vi "Init Dashboard Panel.vi"(8 "error in (no error)":errorcluster, 11 "SB App in":refnum<class "SB App.lvclass">) -> (0 "error out":errorcluster, 3 "SB App out":refnum<class "SB App.lvclass">)   [LabVIEW 2020, in "SB App.lvlib" / "SB App.lvclass"]
uses:
  SB App.lvclass
  Dashboard Panel/Dashboard Panel.lvclass
  C:/Program Files (x86)/National Instruments/LabVIEW 2020/vi.lib/IlluminatedG/IG OOPanel/OOPanel/Panel/Panel.lvclass
  SB App.lvclass/SB App.ctl
  <vilib>/IlluminatedG/IG OOPanel/OOPanel/Manager/Manager.lvclass
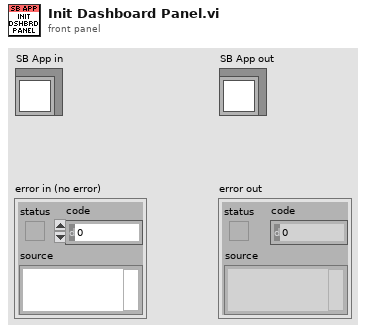
[diagram p1: front panel]
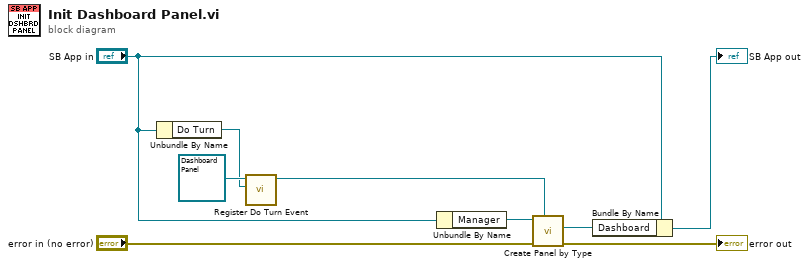
[diagram p0: block diagram]
diagram:
  n1 = Unbundle By Name("SB App in") -> ("Do Turn"=w5:refnum<user-event>)
  n2 = call "Register Do Turn Event.vi"("Do Turn"=w5, "Dashboard Panel in"=refnum<class "Dashboard Panel.lvclass"> refnum ("SB App.lvlib:Dashboard Panel.lvclass")) -> ("Dashboard Panel out"=w4:refnum<class "Dashboard Panel.lvclass">)  [unwired: 8 in, 1 out]
  n3 = Unbundle By Name("SB App in") -> ("Manager"=w9:refnum<class "Manager.lvclass">)
  n4 = call <vilib>:"Create Panel by Type.vi"("Panel Type"=w4, "error in (no error)"="error in (no error)", "Manager in"=w9) -> ("error out"=→"error out":errorcluster, "Panel"=w2:refnum<class "Dashboard Panel.lvclass">)  [unwired: 6 in, 1 out]
  n5 = Bundle By Name(cluster="SB App in", "Dashboard"=w2) -> (→"SB App out":refnum<class "SB App.lvclass">)
